vi "Drive PID.vi"(11 "Process Variable":dbl format="%.2f") -> (3 "Output":dbl format="%.2f")   [LabVIEW 2012]
uses:
  <vilib>/addons/control/pid/NI_PID_pid.lvlib
  <vilib>/addons/control/pid/pid.llb/PID (DBL).vi
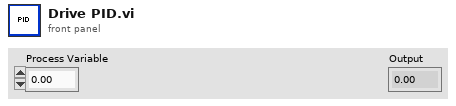
[diagram p1: front panel]
types:
  T1 = cluster{"proportional gain (Kc)":dbl, "integral time (Ti, min)":dbl, "derivative time (Td, min)":dbl}
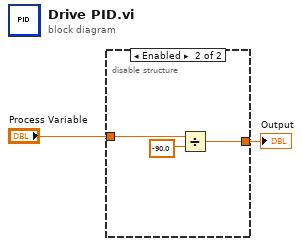
[diagram p0: block diagram]
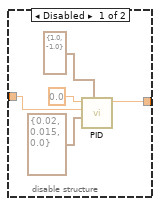
[diagram p2: hidden frame]
diagram:
  n1 = disable-structure shown="Enabled" {
    disable-tunnel: "Process Variable" -> [w5 w10]
    disable-tunnel: [w3 w8] -> w1
    frame Disabled {
      n2 = call-poly <vilib>:"PID.vi"("output range"=cluster{"output high":dbl, "output low":dbl} {"output high"=1.0, "output low"=-1.0}, "PID gains"=T1 {"proportional gain (Kc)"=0.02, "integral time (Ti, min)"=0.015, "derivative time (Td, min)"=0.0}, "process variable"=w5, "setpoint"=0.0) -> ("output"=w3:dbl)  [unwired: 6 in, 1 out]
    }
    frame Enabled {
      n3 = Divide(x=w10, y=-90.0) -> (x/y=w8:dbl)
    }
  }
  "Output" <- w1
